vi "Add Sub Exports.vi"(0 "NSIS_Installer in":refnum<class "Compound_Installer.lvclass">, 5 "SubExport":refnum<class "Export.lvclass">, 11 "error in (no error)":errorcluster) -> (4 "NSIS_Installer out":refnum<class "Compound_Installer.lvclass">, 15 "error out":errorcluster)   [LabVIEW 2017, in "CL_G3_VIComponentBuilder.lvlib" / "Compound_Installer.lvclass"]
doc: "Adds a sub export to the subinstaller lookup table"
uses:
  Compound_Installer.lvclass
  Exports/Export.lvclass
  Compound_Installer.lvclass/Compound_Installer.ctl
  Exports/Export.lvclass/Export.ctl
  Exports/Accessors/Read unique Name.vi
  Accessors/Read Sub Exports.vi
  Accessors/Write Sub Exports.vi
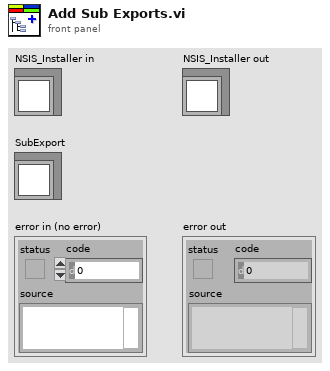
[diagram p1: front panel]
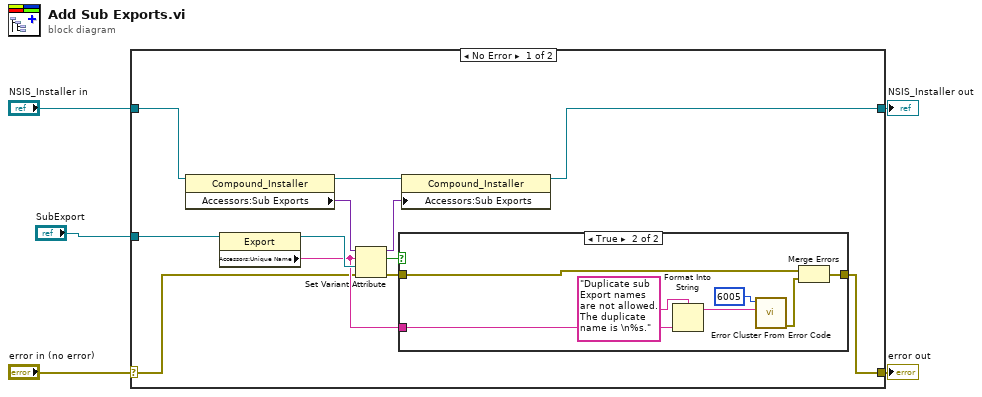
[diagram p0: block diagram]
diagram:
  n1 = case shown="No Error" "error in (no error)" {
    selector: "error in (no error)" -> [w8 w27]
    tunnel: [w7 w27] -> w4
    tunnel: [w9 w26] -> w2
    tunnel: "NSIS_Installer in" -> [w10 w26]
    tunnel: "SubExport" -> [w6 _]
    frame No Error {
      n2 = property class="Compound_Installer"(reference=w10) -> (reference out=w17:refnum<class "Compound_Installer.lvclass">, "Accessors:Sub Exports"=w16:variant)  [unwired: 1 in, 1 out]
      n3 = property class="Export"(reference=w6) -> (reference out=w15:refnum<class "Export.lvclass">, "Accessors:Unique Name"=w11:string)  [unwired: 1 in, 1 out]
      n4 = Set Variant Attribute(Variant=w16, name=w11, value=w15, error in=w8) -> (Variant out=w14:variant, replaced=w13:bool, error out=w12:errorcluster)
      n5 = case shown="True" w13 {
        tunnel: w12 -> [w18 w25]
        tunnel: w11 -> [_ w22]
        tunnel: [w18 w19] -> w7
        frame False {
        }
        frame True {
          n6 = Format Into String(format string="Duplicate sub Export names are not allowed. The duplicate name is \n%s.", w22) -> (resulting string=w21:string)  [unwired: 2 in, 1 out]
          n7 = call <vilib>:"Error Cluster From Error Code.vi"("error message (\"\")"=w21, "error code (0)"=6005) -> ("error out"=w24:errorcluster)  [unwired: 7 in]
          n8 = Merge Errors(w25, w24) -> (w19:errorcluster)
        }
      }
      n9 = property class="Compound_Installer"(reference=w17, "Accessors:Sub Exports"=w14) -> (reference out=w9:refnum<class "Compound_Installer.lvclass">)  [unwired: 1 in, 1 out]
    }
    frame Error {
    }
  }
  "error out" <- w4
  "NSIS_Installer out" <- w2
